vi "Format Attribute.vi"(5 "Attribute Names":string[](array[string]), 6 "Indent":i32, 7 "Attribute Values":variant[](array[variant]), 11 "JSON in":refnum<class "JSON.lvclass">) -> (3 "JSON out":refnum<class "JSON.lvclass">, 4 "Attr Strings":string[](array[string]))   [LabVIEW 2019, in "JSON.lvlib" / "JSON.lvclass"]
uses:
  <vilib>/gpm_packages/@cs/persistence/source/JSON/JSON.lvclass
  1e632909-4be0-42e0-ac58-6dd2f79ca7e1.vi
  <vilib>/JDP Science/JSONtext/Variant to JSON Text.vi
  <vilib>/JDP Science/JSONtext/Set Item.vi
  <vilib>/JDP Science/JSONtext/LVClass Serializer/JSONtext LVClass Serializer.lvclass
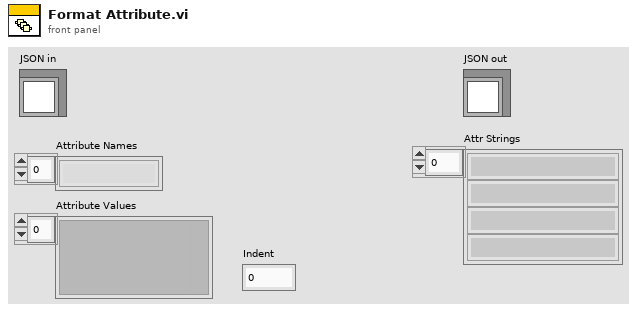
[diagram p1: front panel]
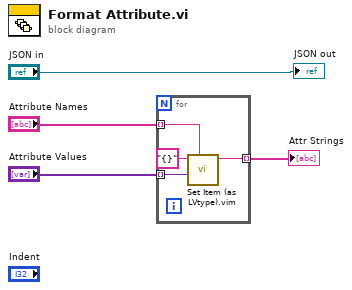
[diagram p0: block diagram]
diagram:
  n1 = for {
    tunnel: "Attribute Values" -> [w8] mode=indexing
    tunnel: "Attribute Names" -> [w7] mode=indexing
    tunnel: [w6] -> w2 mode=indexing
    n2 = call "Set Item (as LVtype).vim"("Object (or Item) Path"=w7, "Anything"=w8, "JSON"="{}") -> ("<JSON>"=w6:string)  [unwired: 5 in, 2 out]
  }
  "Attr Strings" <- w2
  "JSON out" <- "JSON in"
